vi "Anti_deadband_FB_Hawe.vi"(1 "x":sgl) -> (0 "y":sgl)   [LabVIEW 2017]
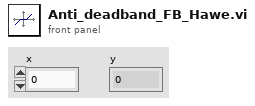
[diagram p1: front panel]
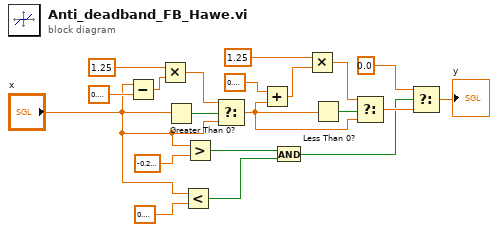
[diagram p0: block diagram]
diagram:
  n1 = Subtract(x="x", y=sgl 0.2 ("single precision float")) -> (x-y=w12:sgl)
  n2 = Multiply(x=sgl 1.25 ("single precision float"), y=w12) -> (x*y=w10:sgl)
  n3 = Greater Than 0?(x="x") -> (x > 0?=w16:bool)
  n4 = Less?(x="x", y=sgl 0.2 ("single precision float")) -> (x < y?=w4:bool)
  n5 = Greater?(x="x", y=sgl -0.2 ("single precision float")) -> (0:w5:bool)
  n6 = Select(t=w10, s=w16, f="x") -> (s? t:f=w9:sgl)
  n7 = Add(x=sgl 0.2 ("single precision float"), y=w9) -> (x+y=w8:sgl)
  n8 = And(x=w5, y=w4) -> (x .and. y?=w6:bool)
  n9 = Multiply(x=sgl 1.25 ("single precision float"), y=w8) -> (x*y=w7:sgl)
  n10 = Less Than 0?(x=w9) -> (x < 0?=w17:bool)
  n11 = Select(t=w7, s=w17, f=w9) -> (s? t:f=w18:sgl)
  n12 = Select(t=sgl 0.0, s=w6, f=w18) -> (s? t:f=→"y":sgl)
